vi "_PC_MS_SubVI displayIonData.vi"(7 "plotName":string, 8 "error in (no error)":errorcluster, 9 "wfmGraph":refnum<vi>, 10 "ionSigInfo":T1) -> (0 "error out":errorcluster)   [LabVIEW 2018]
uses:
  <vilib>/Analysis/baseanly.llb/Mean (DBL).vi
  <vilib>/Analysis/NI_AALBase.lvlib
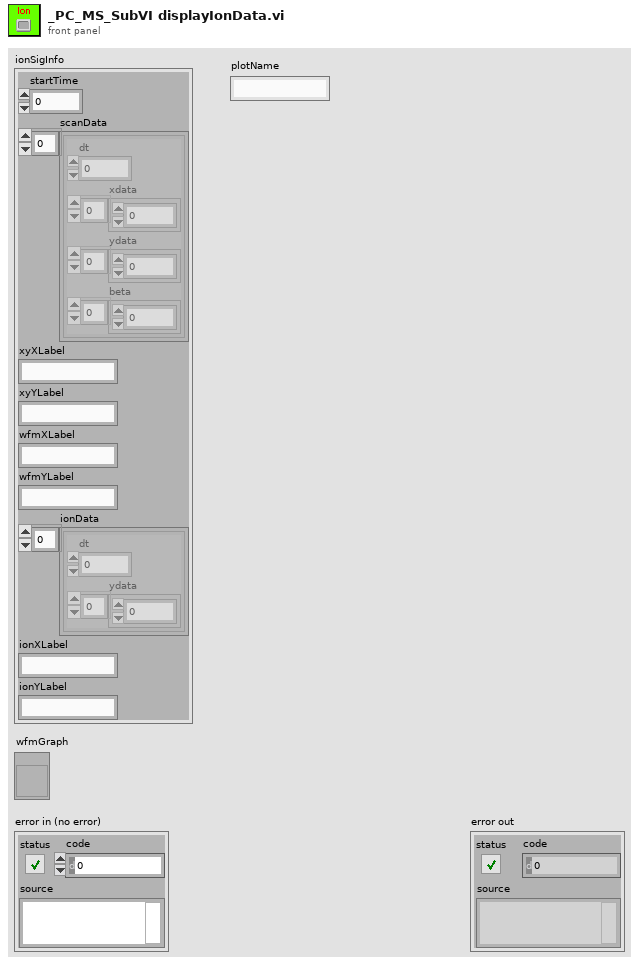
[diagram p1: front panel]
types:
  T1 = cluster{"startTime":dbl, "scanData":cluster{"dt":dbl, "xdata":dbl[], "ydata":sgl[], "beta":dbl[]}[], "xyXLabel":string, "xyYLabel":string, "wfmXLabel":string, "wfmYLabel":string, "ionData":cluster{"dt":dbl, "ydata":sgl[]}[], "ionXLabel":string, "ionYLabel":string}
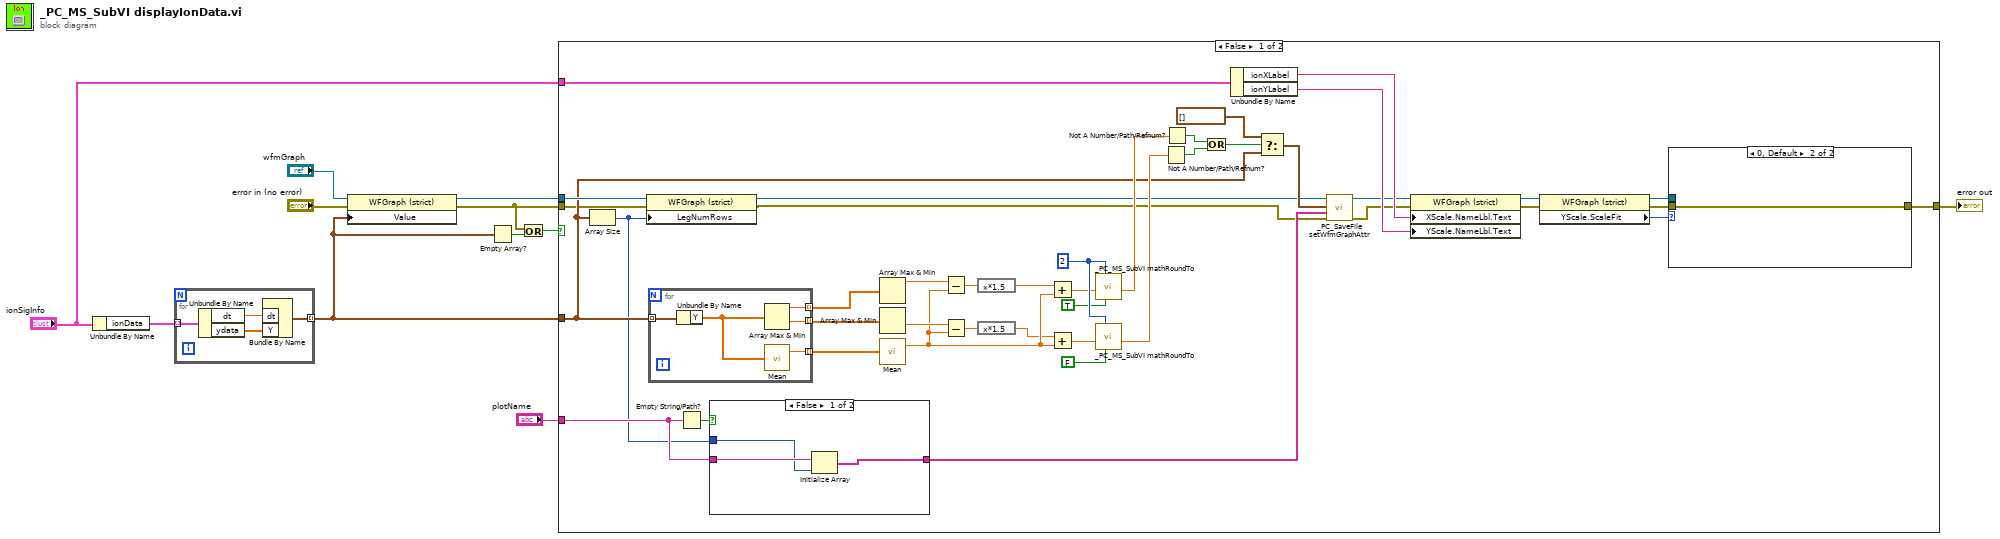
[diagram p0: block diagram]
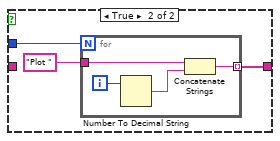
[diagram p2: hidden frame]
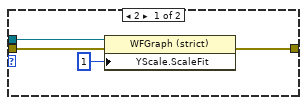
[diagram p3: hidden frame]
diagram:
  n1 = Unbundle By Name("ionSigInfo") -> ("ionData"=w3:cluster{"dt":dbl, "ydata":sgl[]}[])
  n2 = for {
    tunnel: w3 -> [w15] mode=indexing
    tunnel: [w12] -> w2 mode=indexing
    n3 = Unbundle By Name(w15) -> ("dt"=w14:dbl, "ydata"=w13:sgl[])
    n4 = Bundle By Name("dt"=w14, "Y"=w13) -> (w12:waveform(sgl))  [unwired: 1 in]
  }
  n5 = property class="WFGraph (strict)"(reference="wfmGraph", error in="error in (no error)", "Value"=w2) -> (reference out=w10:refnum<vi>, error out=w5:errorcluster)
  n6 = Empty Array?(array=w2) -> (empty?=w7:bool)
  n7 = Or(x=w5, y=w7) -> (x .or. y?=w6:bool)
  n8 = case shown="False" w6 {
    tunnel: [w35 w78] -> w11
    tunnel: w10 -> [w38 _]
    tunnel: w2 -> [w32 _]
    tunnel: "plotName" -> [w30 _]
    tunnel: w5 -> [w31 w78]
    tunnel: "ionSigInfo" -> [w24 _]
    frame False {
      w57 = 2 ("Digit")
      n9 = Array Size(array=w32) -> (size(s)=w28:i32)
      n10 = property class="WFGraph (strict)"(reference=w38, error in=w31, "LegNumRows"=w28) -> (reference out=w17:refnum<vi>, error out=w16:errorcluster)
      n11 = for {
        tunnel: [w77] -> w55 mode=indexing
        tunnel: [w76] -> w56 mode=indexing
        tunnel: w32 -> [w74] mode=indexing
        tunnel: [w75] -> w54 mode=indexing
        n12 = Unbundle By Name(w74) -> ("Y"=w73:sgl[])
        n13 = Array Max & Min(array=w73) -> (max value=w76:sgl, min value=w77:sgl)  [unwired: 2 out]
        n14 = call-poly <vilib>:"Mean.vi"("X"=w73) -> ("mean"=w75:dbl)  [unwired: 1 out]
      }
      n15 = Empty String/Path?(string/path=w30) -> (empty?=w29:bool)
      n16 = case shown="False" w29 {
        tunnel: w28 -> [w59 w63]
        tunnel: [w58 w61] -> w20
        tunnel: w30 -> [w60 _]
        frame False {
          n17 = Initialize Array(w60, w59) -> (w58:string[])
        }
        frame True {
          n18 = for {
            N: w63 -> [_]
            tunnel: "Plot " -> [w65]
            tunnel: [w64] -> w61 mode=indexing
            i -> [w66]
            n19 = Number To Decimal String(number=w66) -> (decimal integer string=w67:string)  [unwired: 1 in]
            n20 = Concatenate Strings(w65, w67) -> (w64:string)
          }
        }
      }
      n21 = Array Max & Min(array=w56) -> (max value=w53:sgl)  [unwired: 3 out]
      n22 = Array Max & Min(array=w55) -> (min value=w52:sgl)  [unwired: 3 out]
      n23 = call-poly <vilib>:"Mean.vi"("X"=w54) -> ("mean"=w49:dbl)  [unwired: 1 out]
      n24 = Subtract(x=w53, y=w49) -> (x-y=w51:dbl)
      n25 = Subtract(x=w52, y=w49) -> (x-y=w50:dbl)
      n26 = expression code="x*1.5"(w51) -> (w47:dbl)
      n27 = expression code="x*1.5"(w50) -> (w48:dbl)
      n28 = Add(x=w47, y=w49) -> (x+y=w46:dbl)
      n29 = Add(x=w48, y=w49) -> (x+y=w45:dbl)
      n30 = call "_PC_MS_SubVI mathRoundTo.vi"("Up/Down"=TRUE, "Digit"=w57, "Numeric"=w46) -> ("Round to"=w34:dbl)  [unwired: 8 in]
      n31 = call "_PC_MS_SubVI mathRoundTo.vi"("Up/Down"=FALSE, "Digit"=w57, "Numeric"=w45) -> ("Round to"=w33:dbl)  [unwired: 8 in]
      n32 = Not A Number/Path/Refnum?(number/path/refnum=w33) -> (NaN/Path/Refnum?=w39:bool)
      n33 = Not A Number/Path/Refnum?(number/path/refnum=w34) -> (NaN/Path/Refnum?=w40:bool)
      n34 = Or(x=w40, y=w39) -> (x .or. y?=w37:bool)
      n35 = Unbundle By Name(w24) -> ("ionXLabel"=w23:string, "ionYLabel"=w22:string)
      n36 = Select(t=waveform(sgl)[] [], s=w37, f=w32) -> (s? t:f=w21:waveform(sgl)[])
      n37 = call "_PC_SaveFile setWfmGraphAttr.vi"("error in (no error)"=w16, "plotName"=w20, "plotValue"=w21, "graph in"=w17) -> ("error out"=w18:errorcluster, "graph out"=w19:refnum<vi>)  [unwired: 6 in]
      n38 = property class="WFGraph (strict)"(reference=w19, error in=w18, "XScale.NameLbl.Text"=w23, "YScale.NameLbl.Text"=w22) -> (reference out=w26:refnum<vi>, error out=w25:errorcluster)
      n39 = property class="WFGraph (strict)"(reference=w26, error in=w25) -> (reference out=w42:refnum<vi>, error out=w36:errorcluster, "YScale.ScaleFit"=w41:u8)
      n40 = case shown="0, Default" w41 {
        tunnel: [w71 w72] -> w35
        tunnel: w42 -> [w70 _]
        tunnel: w36 -> [w68 w72]
        frame 2 {
          n41 = property class="WFGraph (strict)"(reference=w70, error in=w68, "YScale.ScaleFit"=u8 1 ("Y Scale.Scale Fit")) -> (error out=w71:errorcluster)  [unwired: 1 out]
        }
        frame 0, Default {
        }
      }
    }
    frame True {
    }
  }
  "error out" <- w11
